vi "Export - Main.vi"(8 "error in (no error)":errorcluster, 11 "Device Item Ref in":T19 format="%.0x") -> (0 "error out":errorcluster, 3 "Import/Export Data":T1 {"Tx Packets"."Tx Packet Data"."threadOptions"."pclDecimation" max=16 step=1; "Tx Packets"."Tx Packet Data"."threadOptions"."loopPeriod" max=16 step=1; "Tx Packets"."Tx Packet Data"."threadOptions"."targetPriority" min=-2 max=16 step=1; "Tx Packets"."Tx Packet Data"."threadOptions"."targetProcessor" min=-2 max=16 step=1; "Tx Packets"."Tx Packet Data"."Endianness" items=["big-endian"=0, "little-endian"=2]; "Rx Packets"."Rx Packet Data"."targetPriority" min=-2 max=16 step=1; "Rx Packets"."Rx Packet Data"."targetProcessor" min=-2 max=16 step=1; "Rx Packets"."Rx Packet Data"."Endianness" items=["big-endian"=0, "little-endian"=2]})   [LabVIEW 2019, in "UDP-Custom-Device System Explorer.lvlib"]
uses:
  UDP-Custom-Device System Explorer.lvlib
  <vilib>/NI VeriStand/Custom Device API/Custom Device Item Ref.ctl
  Types/XML - New/ImpExp - Data.ctl
  Types/XML - New/ImpExp - Main Data.ctl
  <vilib>/NI VeriStand/Custom Device API/Custom Device Item Info.ctl
  Types/XML - New/ImpExp - Rx Packets Data.ctl
  Types/XML - New/ImpExp - Rx Packet Data.ctl
  Shared/Types/Shared - Channel Data Type.ctl
  Shared/Types/Shared - Buffered.PacketInfo.ctl
  Shared/Types/Shared - Pointer Encoding.ctl
  Shared/Types/Shared - Receive Buffer Options.ctl
  Shared/Types/Shared - Transmit Buffer Options.ctl
  Shared/Types/Shared - New Data Options.ctl
  Shared/Types/Shared - Thread Management.ctl
  Types/XML - New/ImpExp - Tx Packets Data.ctl
  Types/XML - New/ImpExp - Tx Packet Data.ctl
  Shared/Types/Shared - Transmit Flag Options.ctl
  Shared/Types/Shared - Transmit Echo Options.ctl
  Types/Threading/Thread Configuration.ctl
  Types/Threading/Thread Sync Reference.ctl
  Property Accessors/Main Accessors.lvlib
  <vilib>/NI VeriStand/Custom Device API/Custom Device API.lvlib
  Shared/UDP-Custom-Device Shared.lvlib
  <vilib>/NI VeriStand/Custom Device Tools/Custom Device Utility Library/Custom Device Utility Library.lvlib
panel:
  out "Controller Path":string
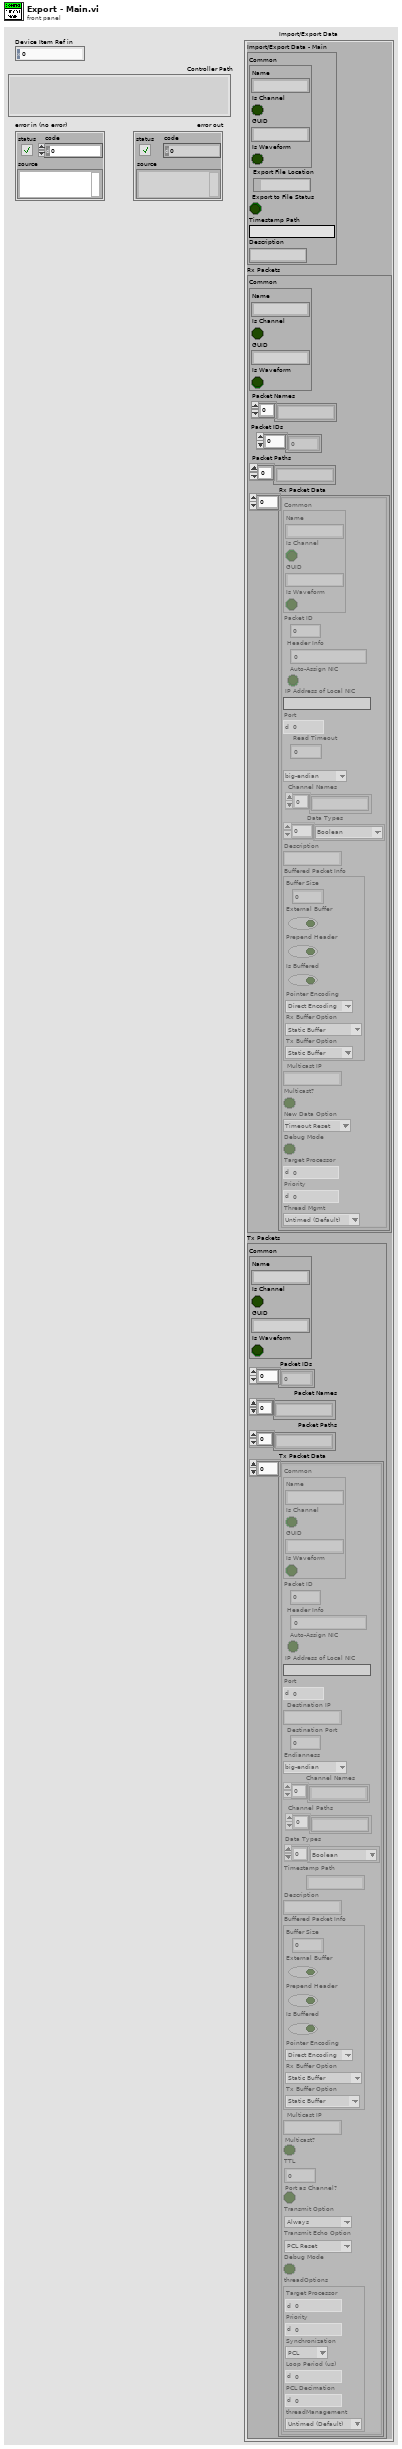
[diagram p1: front panel]
types:
  T1 = typedef "UDP-Custom-Device System Explorer.lvlib/ImpExp - Data.ctl" = cluster{"Import/Export Data - Main":T2, "Rx Packets":T4, "Tx Packets":T13}
  T2 = typedef "UDP-Custom-Device System Explorer.lvlib/ImpExp - Main Data.ctl" = cluster{"Common":T3, "Export File Location":path, "Export to File Status":bool, "Timestamp Path":string, "Description":string}
  T3 = typedef "Custom Device API.lvlib/Custom Device Item Info.ctl" = cluster{"Name":string, "Is Channel":bool, "GUID":string, "Is Waveform":bool}
  T4 = typedef "UDP-Custom-Device System Explorer.lvlib/ImpExp - Rx Packets Data.ctl" = cluster{"Common":T3, "Packet Names":string[], "Packet IDs":i32[], "Packet Paths":string[], "Rx Packet Data":T5[]}
  T5 = typedef "UDP-Custom-Device System Explorer.lvlib/ImpExp - Rx Packet Data.ctl" = cluster{"Common":T3, "Packet ID":i32, "Header Info":u32, "Auto-Assign NIC":bool, "IP Address of Local NIC":string, "Port":u16, "Read Timeout":i32, "Endianness":u16, "Channel Names":string[], "Data Types":T6[], "Description":string, "Buffered Packet Info":T7, "Multicast IP":string, "Multicast?":bool, "New Data Option":T11, "Debug Mode":bool, "targetProcessor":i8, "targetPriority":i16, "Thread Mgmt":T12}
  T6 = typedef "UDP-Custom-Device Shared.lvlib/Shared - Channel Data Type.ctl" = enum16{"Boolean", "Single", "Double", "I8", "I16", "I32", "I64", "U8", "U16", "U32", "U64"}
  T7 = typedef "UDP-Custom-Device Shared.lvlib/Shared - Buffered.PacketInfo.ctl" = cluster{"Buffer Size":i32, "External Buffer":bool, "Prepend Header":bool, "Is Buffered":bool, "Pointer Encoding":T8, "Rx Buffer Option":T9, "Tx Buffer Option":T10}
  T8 = typedef "UDP-Custom-Device Shared.lvlib/Shared - Pointer Encoding.ctl" = enum16{"Direct Encoding", "Conversion Encoding"}
  T9 = typedef "UDP-Custom-Device Shared.lvlib/Shared - Receive Buffer Options.ctl" = enum16{"Static Buffer", "Circular Buffer", "Circular Buffer + Size", "Internal Cache", "Internal Cache + Size", "Ping Pong", "Ping Pong + Size"}
  T10 = typedef "UDP-Custom-Device Shared.lvlib/Shared - Transmit Buffer Options.ctl" = enum16{"Static Buffer", "FIFO Buffer", "FIFO Buffer + Port"}
  T11 = typedef "UDP-Custom-Device Shared.lvlib/Shared - New Data Options.ctl" = enum16{"Timeout Reset", "Counter"}
  T12 = typedef "UDP-Custom-Device Shared.lvlib/Shared - Thread Management.ctl" = enum16{"Untimed (Default)", "Timed (High Priority)"}
  T13 = typedef "UDP-Custom-Device System Explorer.lvlib/ImpExp - Tx Packets Data.ctl" = cluster{"Common":T3, "Packet IDs":i32[], "Packet Names":string[], "Packet Paths":string[], "Tx Packet Data":T14[]}
  T14 = typedef "UDP-Custom-Device System Explorer.lvlib/ImpExp - Tx Packet Data.ctl" = cluster{"Common":T3, "Packet ID":i32, "Header Info":u32, "Auto-Assign NIC":bool, "IP Address of Local NIC":string, "Port":u16, "Destination IP":string, "Destination Port":u16, "Endianness":u16, "Channel Names":string[], "Channel Paths":string[], "Data Types":T6[], "Timestamp Path":string, "Description":string, "Buffered Packet Info":T7, "Multicast IP":string, "Multicast?":bool, "TTL":u16, "Port as Channel?":bool, "Transmit Option":T15, "Transmit Echo Option":T16, "Debug Mode":bool, "threadOptions":T17}
  T15 = typedef "UDP-Custom-Device Shared.lvlib/Shared - Transmit Flag Options.ctl" = enum16{"Always", "One-Shot", "Toggle"}
  T16 = typedef "UDP-Custom-Device Shared.lvlib/Shared - Transmit Echo Options.ctl" = enum16{"PCL Reset", "Counter", "Mirror"}
  T17 = typedef "UDP-Custom-Device System Explorer.lvlib/Thread Configuration.ctl" = cluster{"targetProcessor":i8, "targetPriority":i16, "Synchronization":T18, "loopPeriod":u32, "pclDecimation":u16, "threadManagement":T12}
  T18 = typedef "UDP-Custom-Device System Explorer.lvlib/Thread Sync Reference.ctl" = enum16{"PCL", "Async"}
  T19 = typedef "Custom Device API.lvlib/Custom Device Item Ref.ctl" = u64
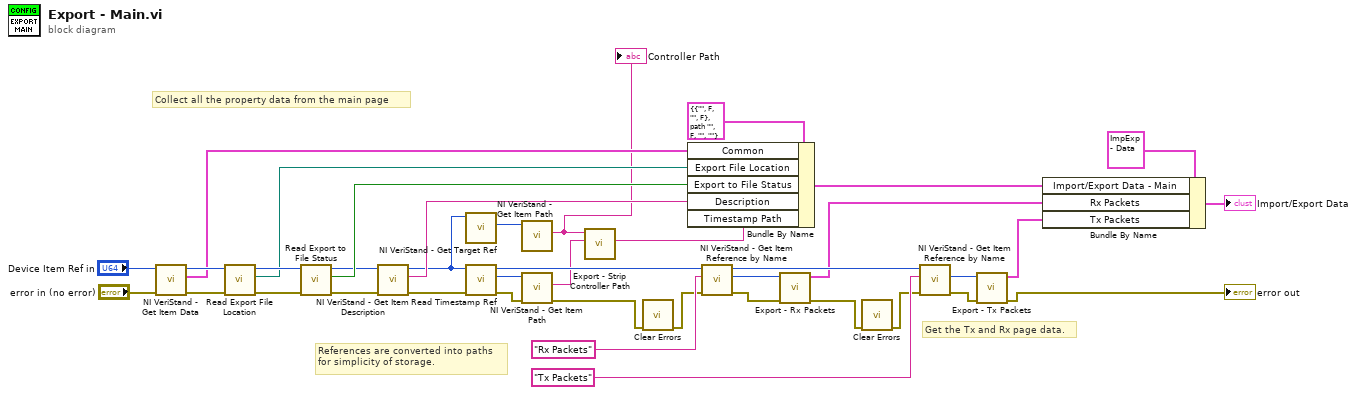
[diagram p0: block diagram]
diagram:
  # "References are converted into paths\nfor simplicity of storage."
  # "Get the Tx and Rx page data."
  # "Collect all the property data from the main page"
  n1 = call <vilib>:"NI VeriStand - Get Item Data.vi"("error in (no error)"="error in (no error)", "Item Ref in"="Device Item Ref in") -> ("error out"=w32:errorcluster, "Item Info"=w29:T3, "Item Ref out"=w34:T19)  [unwired: 6 in, 1 out]
  n2 = call "Read Export File Location.vi"("error in (no error)"=w32, "Node Ptr"=w34) -> ("error out"=w39:errorcluster, "Export File Location"=w28:path, "Node Ptr out"=w38:T19)  [unwired: 7 in]
  n3 = call "Read Export to File Status.vi"("error in (no error)"=w39, "Node Ptr"=w38) -> ("error out"=w11:errorcluster, "Export to File Status"=w27:bool, "Node Ptr out"=w8:T19)  [unwired: 7 in]
  n4 = call <vilib>:"NI VeriStand - Get Item Description.vi"("error in (no error)"=w11, "Item Ref in"=w8) -> ("error out"=w10:errorcluster, "Description"=w7:string, "Item Ref out"=w6:T19)  [unwired: 6 in, 1 out]
  n5 = call <vilib>:"NI VeriStand - Get Target Ref.vi"("Item Ref in"=w6) -> ("Target Ref"=w9:T19)  [unwired: 7 in, 3 out]
  n6 = call "Read Timestamp Ref.vi"("error in (no error)"=w10, "Node Ptr"=w6) -> ("error out"=w36:errorcluster, "Timestamp Ref"=w37:T19, "Node Ptr out"=w25:T19)  [unwired: 7 in]
  n7 = call <vilib>:"NI VeriStand - Get Item Path.vi"("Item Ref in"=w9) -> ("Path"=w3:string)  [unwired: 7 in, 3 out]
  "Controller Path" <- w3
  n8 = call <vilib>:"NI VeriStand - Get Item Path.vi"("error in (no error)"=w36, "Item Ref in"=w37) -> ("error out"=w13:errorcluster, "Path"=w5:string)  [unwired: 6 in, 2 out]
  n9 = call "Export - Strip Controller Path.vi"("Channel Path"=w5, "Controller Path"=w3) -> ("Stripped Path"=w4:string)  [unwired: 8 in, 1 out]
  n10 = call <vilib>:"Clear Errors.vi"("error in (no error)"=w13) -> ("error out"=w12:errorcluster)  [unwired: 5 in, 1 out]
  n11 = Bundle By Name(cluster=T2 {"Common"={"Name"="", "Is Channel"=FALSE, "GUID"="", "Is Waveform"=FALSE}, "Export File Location"=path "", "Export to File Status"=FALSE, "Timestamp Path"="", "Description"=""} ("Import/Export Data - Main"), "Common"=w29, "Export File Location"=w28, "Export to File Status"=w27, "Description"=w7, "Timestamp Path"=w4) -> (w30:T2)
  n12 = call <vilib>:"NI VeriStand - Get Item Reference by Name.vi"("error in (no error)"=w12, "Item Name"="Rx Packets" ("Section Name"), "Parent Ref in"=w25) -> ("error out"=w18:errorcluster, "Item Ref"=w20:T19, "Parent Ref out"=w23:T19)  [unwired: 5 in, 1 out]
  n13 = call "Export - Rx Packets.vi"("error in (no error)"=w18, "Device Item Ref in"=w20) -> ("error out"=w2:errorcluster, "Rx Packets"=w19:T4)  [unwired: 8 in]
  n14 = call <vilib>:"Clear Errors.vi"("error in (no error)"=w2) -> ("error out"=w1:errorcluster)  [unwired: 5 in, 1 out]
  n15 = call <vilib>:"NI VeriStand - Get Item Reference by Name.vi"("error in (no error)"=w1, "Item Name"="Tx Packets" ("Section Name"), "Parent Ref in"=w23) -> ("error out"=w15:errorcluster, "Item Ref"=w17:T19)  [unwired: 5 in, 2 out]
  n16 = call "Export - Tx Packets.vi"("error in (no error)"=w15, "Device Item Ref in"=w17) -> ("error out"=→"error out":errorcluster, "Tx Packets"=w16:T13)  [unwired: 8 in]
  n17 = Bundle By Name(cluster=T1 {"Import/Export Data - Main"={"Common"={"Name"="", "Is Channel"=FALSE, "GUID"="", "Is Waveform"=FALSE}, "Export File Location"=path "", "Export to File Status"=FALSE, "Timestamp Path"="", "Description"=""}, "Rx Packets"={"Common"={"Name"="", "Is Channel"=FALSE, "GUID"="", "Is Waveform"=FALSE}, "Packet Names"=[], "Packet IDs"=[], "Packet Paths"=[], "Rx Packet Data"=[]}, "Tx Packets"={"Common"={"Name"="", "Is Channel"=FALSE, "GUID"="", "Is Waveform"=FALSE}, "Packet IDs"=[], "Packet Names"=[], "Packet Paths"=[], "Tx Packet Data"=[]}} ("Import/Export Data"), "Import/Export Data - Main"=w30, "Rx Packets"=w19, "Tx Packets"=w16) -> (→"Import/Export Data":T1)
